vi "Get Supported Frequency Range.vi"(0 "Instrument Model":string, 5 "Instrument Name":string, 11 "error in":errorcluster) -> (4 "Maximum Frequency":dbl, 6 "Minmum Frequency":dbl, 15 "error out":errorcluster)   [LabVIEW 2023, in "RFFixtureCharact.Public.lvlib" / "Scalar Path.lvclass"]
uses:
  Scalar Path.lvclass
  <vilib>/nisyscfg/Close (Resources).vi
  <vilib>/nisyscfg/Close (Filter).vi
  <vilib>/nisyscfg/Close (System).vi
  Scalar Path.lvclass/Scalar Path.ctl
  <vilib>/nisyscfg/nisyscfg.lvlib
  <resource>/objmgr/niflexrioatomicsae.rc
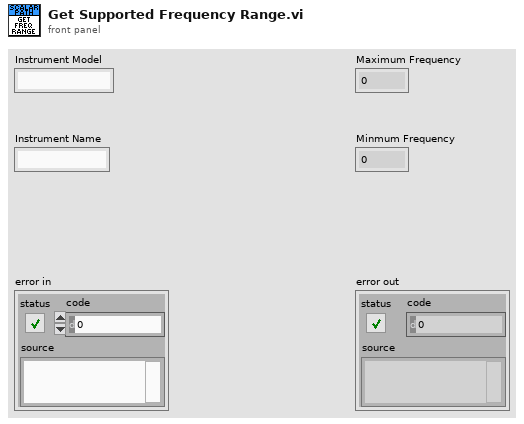
[diagram p1: front panel]
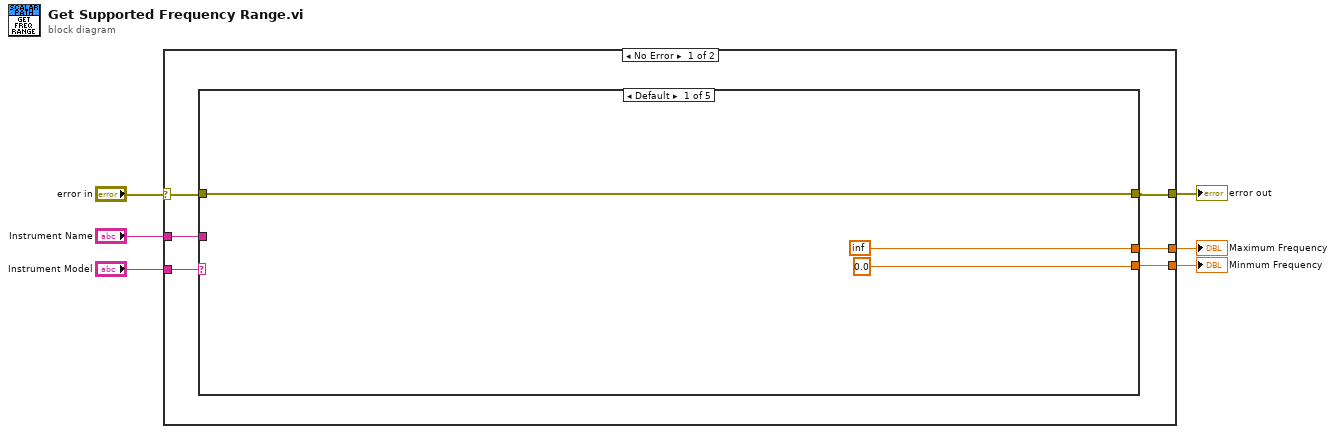
[diagram p0: block diagram]
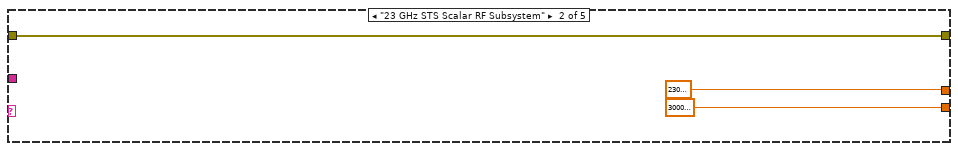
[diagram p2: hidden frame]
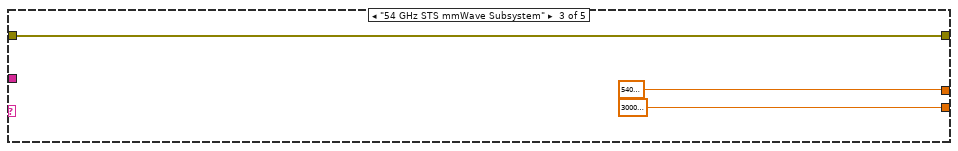
[diagram p3: hidden frame]
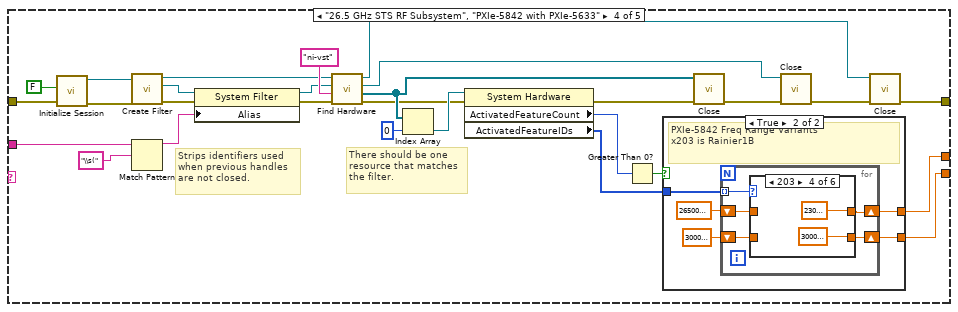
[diagram p4: hidden frame]
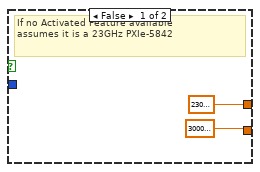
[diagram p5: hidden frame]
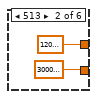
[diagram p7: hidden frame]
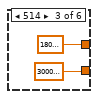
[diagram p8: hidden frame]
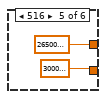
[diagram p9: hidden frame]
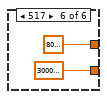
[diagram p10: hidden frame]
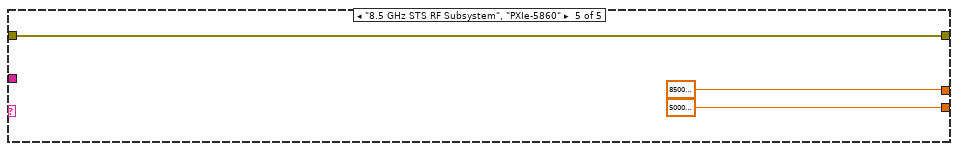
[diagram p11: hidden frame]
diagram:
  n1 = case shown="No Error" "error in" {
    selector: "error in" -> [w12 w77]
    tunnel: [w9 w77] -> w6
    tunnel: "Instrument Model" -> [w11 _]
    tunnel: "Instrument Name" -> [w10 _]
    tunnel: [w8 _] -> w2
    tunnel: [w7 _] -> w1
    frame No Error {
      n2 = case shown="Default" w11 {
        tunnel: [w15 w16 w19 w49 w74] -> w9
        tunnel: [0.0 30000000.0 30000000.0 w48 50000000.0] -> w7
        tunnel: [inf 23000000000.0 54000000000.0 w47 8500000000.0] -> w8
        tunnel: w10 -> [_ _ _ w46 _]
        tunnel: w12 -> [w15 w16 w19 w22 w74]
        frame Default {
        }
        frame "23 GHz STS Scalar RF Subsystem" {
        }
        frame "54 GHz STS mmWave Subsystem" {
        }
        frame "26.5 GHz STS RF Subsystem", "PXIe-5842 with PXIe-5633" {
          # "Strips identifiers used\nwhen previous handles\nare not closed."
          # "There should be one\nresource that matches\nthe filter."
          n3 = call <vilib>:"Initialize Session.vi"("error in (no error)"=w22, "Force Property Refresh (T)"=FALSE) -> ("error out"=w44:errorcluster, "Session out"=w45:refnum<k21>)  [unwired: 8 in]
          n4 = call <vilib>:"Create Filter.vi"("error in (no error)"=w44, "Session in"=w45) -> ("error out"=w38:errorcluster, "Filter out"=w36:refnum<k20>, "Session out"=w35:refnum<k21>)  [unwired: 7 in]
          n5 = Match Pattern(string=w46, regular expression="\\s(") -> (before substring=w27:string)  [unwired: 1 in, 3 out]
          n6 = property class="System Filter"(reference=w36, error in=w38, "Alias"=w27) -> (reference out=w37:refnum<k20>, error out=w39:errorcluster)
          n7 = call <vilib>:"Find Hardware.vi"("error in (no error)"=w39, "Experts"="ni-vst", "Filter in"=w37, "Session in"=w35) -> ("error out"=w30:errorcluster, "Resources out"=w32:refnum<k20>[], "Filter out"=w33:refnum<k20>, "Session out"=w28:refnum<k21>)  [unwired: 4 in]
          n8 = Index Array(array=w32, index=0) -> (element=w31:refnum<k20>)
          n9 = property class="System Hardware"(reference=w31, error in=w30) -> (error out=w29:errorcluster, "ActivatedFeatureCount"=w25:u32, "ActivatedFeatureIDs"=w24:u32[])  [unwired: 1 out]
          n10 = Greater Than 0?(x=w25) -> (x > 0?=w26:bool)
          n11 = case shown="True" w26 {
            tunnel: [23000000000.0 w56] -> w47
            tunnel: [30000000.0 w55] -> w48
            tunnel: w24 -> [_ w54]
            frame False {
              # "If no Activated Feature available\nassumes it is a 23GHz PXIe-5842"
            }
            frame True {
              # "PXIe-5842 Freq Range Variants\nx203 is Rainier1B"
              n12 = for {
                shift-right: [w60] -> w56
                shift-left: 26500000000.0 -> [w61]
                shift-right: [w59] -> w55
                shift-left: 30000000.0 -> [w58]
                tunnel: w54 -> [w57] mode=indexing
                n13 = case shown="203" w57 {
                  tunnel: [w63 12000000000.0 18000000000.0 23000000000.0 26500000000.0 8000000000.0] -> w60
                  tunnel: w61 -> [w63 _ _ _ _ _]
                  tunnel: [w62 30000000.0 30000000.0 30000000.0 30000000.0 30000000.0] -> w59
                  tunnel: w58 -> [w62 _ _ _ _ _]
                  frame Default {
                  }
                  frame 513 {
                  }
                  frame 514 {
                  }
                  frame 515 {
                  }
                  frame 516 {
                  }
                  frame 517 {
                  }
                }
              }
            }
          }
          n14 = call-poly <vilib>:"Close.vi"("error in (no error)"=w29, "Resources in"=w32) -> ("error out"=w34:errorcluster)  [unwired: 9 in]
          n15 = call-poly <vilib>:"Close.vi"("error in (no error)"=w34, "Filter in"=w33) -> ("error out"=w40:errorcluster)  [unwired: 9 in]
          n16 = call-poly <vilib>:"Close.vi"("error in (no error)"=w40, "Session in"=w28) -> ("error out"=w49:errorcluster)  [unwired: 9 in]
        }
        frame "8.5 GHz STS RF Subsystem", "PXIe-5860" {
        }
      }
    }
    frame Error {
    }
  }
  "error out" <- w6
  "Maximum Frequency" <- w2
  "Minmum Frequency" <- w1
